vi "Remove All Aliases.vi"(8 "error in (no error)":errorcluster, 11 "Aliases Ref in":T1 format="%.0x") -> (0 "error out":errorcluster, 3 "Aliases Ref out":T1 format="%.0x")   [LabVIEW 2017, in "Routing and Faulting Scripting.lvlib"]
uses:
  Routing and Faulting Scripting.lvlib
  <vilib>/NI Veristand/Custom Device API/Custom Device Item Ref.ctl
  <vilib>/NI VeriStand/Custom Device API/Custom Device API.lvlib
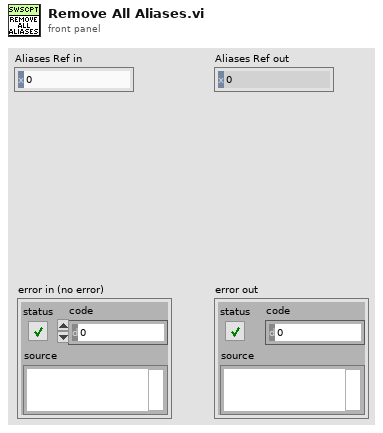
[diagram p1: front panel]
types:
  T1 = typedef "Custom Device API.lvlib/Custom Device Item Ref.ctl" = u64
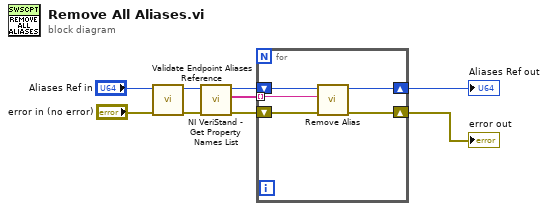
[diagram p0: block diagram]
diagram:
  n1 = call "Validate Endpoint Aliases Reference.vi"("error in (no error)"="error in (no error)", "Endpoint Aliases Ref in"="Aliases Ref in") -> ("error out"=w3:errorcluster, "Endpoint Aliases Ref out"=w1:T1)  [unwired: 8 in]
  n2 = call <vilib>:"NI VeriStand - Get Property Names List.vi"("error in (no error)"=w3, "Item Ref in"=w1) -> ("error out"=w8:errorcluster, "Property Names"=w9:string[], "Item Ref out"=w5:T1)  [unwired: 7 in]
  n3 = for {
    tunnel: w9 -> [w12] mode=indexing
    shift-right: [w10] -> w6
    shift-left: w8 -> [w11]
    shift-right: [w13] -> w4
    shift-left: w5 -> [w14]
    n4 = call "Remove Alias.vi"("error in (no error)"=w11, "Alias"=w12, "Endpoint Aliases Ref in"=w14) -> ("error out"=w10:errorcluster, "Endpoint Aliases Ref out"=w13:T1)  [unwired: 7 in]
  }
  "error out" <- w6
  "Aliases Ref out" <- w4
